vi "ShutdownCleanup AMC and OPC.vi"(8 "error in (no error)":errorcluster, 9 "Array of Variables":refnum<k21>[](array[refnum])) -> ()   [LabVIEW 2019]
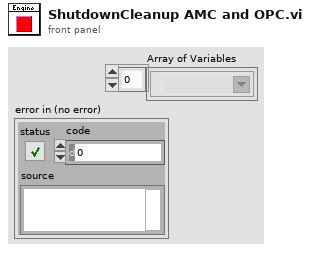
[diagram p1: front panel]
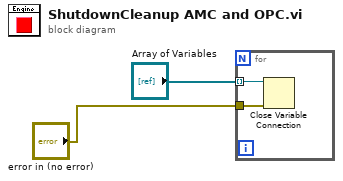
[diagram p0: block diagram]
diagram:
  n1 = for {
    tunnel: "Array of Variables" -> [w4] mode=indexing
    tunnel: "error in (no error)" -> [w3]
    n2 = Close Variable Connection(8:w3, 11:w4) -> ()  [unwired: 1 out]
  }
